vi "test.vi"() -> ()   [LabVIEW 2009]
uses:
  <vilib>/imath/engines/lvmath2/RunTimeEngine/ErrorHandling/NIMS_Finalize Error.vi
  <vilib>/imath/engines/lvmath2/RunTimeEngine/Parser/MC_Version.vi
  <vilib>/imath/engines/lvmath2/RunTimeEngine/NodeEndStatement/NIMS_NodeEndStatement_Output.vi
  <instcachedir>/0/NIMS_NodeEndStatement_Output_B70DDD75627E4997AAE11E9955EDAA25.lvgen/NIMS_NodeEndStatement_Output_B70DDD75627E4997AAE11E9955EDAA25_003.vi
  <instcachedir>/0/NIMS_NodeEndStatement_Output_B70DDD75627E4997AAE11E9955EDAA25.lvgen/NIMS_NodeEndStatement_Output_B70DDD75627E4997AAE11E9955EDAA25_008.vi
  <vilib>/imath/engines/lvmath/Functions/Error Handling/MergeErrorsWrapper.vi
  <vilib>/imathl/engines/lvmath/Functions/Error Handling/Create Error.vi
  <vilib>/imath/engines/lvmath/Functions/Error Handling/MC_Error Cluster From Error Code.vi
  <vilib>/imath/engines/lvmath2/RunTimeEngine/BuiltInFunctions/rand/NIMS_rand(I32).vi
  <vilib>/imath/engines/lvmath2/RunTimeEngine/BuiltInFunctions/rand/NIMS_rand(1,I32).vi
panel:
  out "Map":dbl[][](array[numeric])
  out "Distance No COMPLEX":dbl
  out "FreePath 2":bool
  out "Distance":dbl
  in  "error in":errorcluster
  in  "Size":i32
  out "error out":errorcluster
  out "FreePath":bool
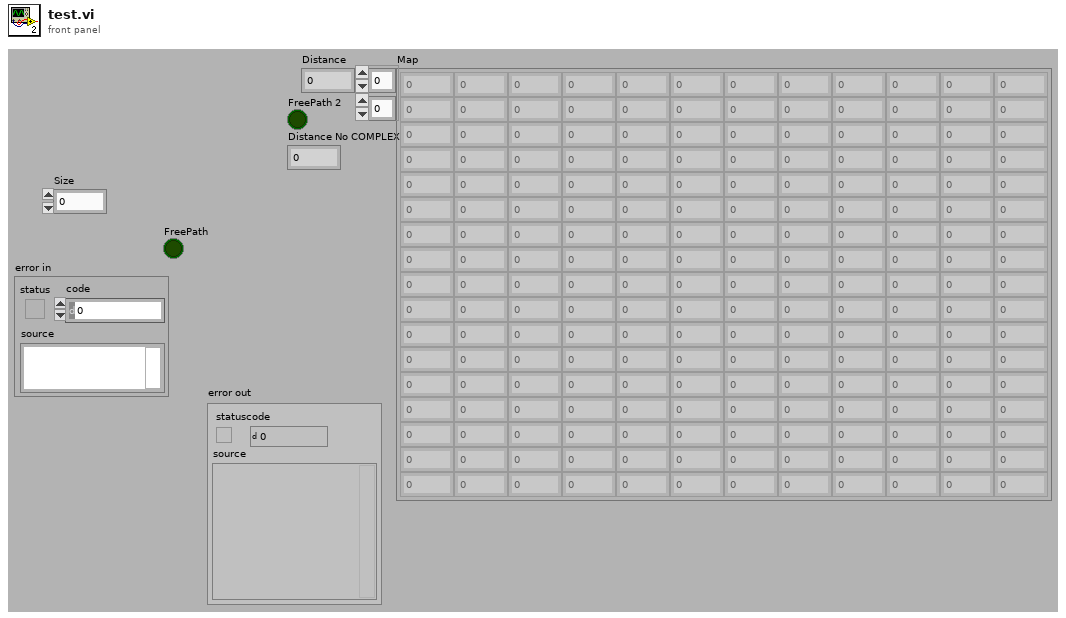
[diagram p1: front panel]
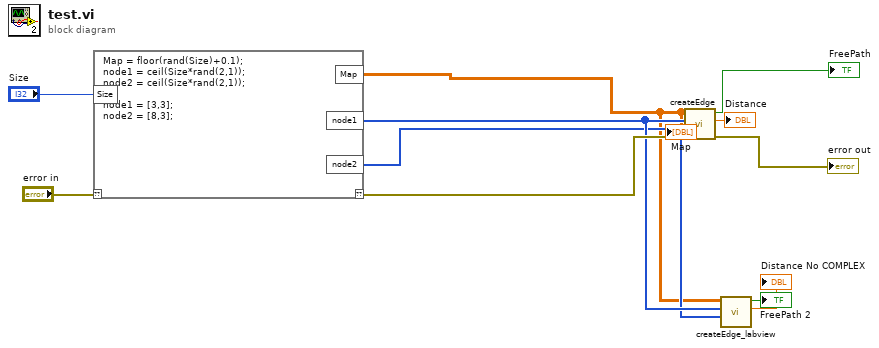
[diagram p0: block diagram]
diagram:
  n1 = mathscript code="Map = floor(rand(Size)+0.1);\nnode1 = ceil(Size*rand(2,1));\nnode2 = ceil(Size*rand(2,1));\n\nnode1 = [3,3];\nnode2 = [8,3];"("??"="error in", "Size"="Size") -> ("??"=w11:errorcluster, "Map"=w1:dbl[][], "node1"=w5:i32[], "node2"=w4:i32[])
  "Map" <- w1
  n2 = call "createEdge.vi"("error in (no error)"=w11, "node 2"=w4, "node1"=w5, "Map"=w1) -> ("error out"=→"error out":errorcluster, "Distance"=→"Distance":dbl, "FreePath"=→"FreePath":bool)  [unwired: 2 in]
  n3 = call "createEdge_labview.vi"("node 2"=w4, "node1"=w5, "Map"=w1) -> ("Distance No COMPLEX"=→"Distance No COMPLEX":dbl, "FreePath"=→"FreePath 2":bool)  [unwired: 7 in]
